vi "DAQ_TDV Meas Configure and Measure.vi"(0 "DAQmx Task In":refnum<k21>, 2 "Execution Settings":T2, 5 "Range and Terminal Settings":T7={"Global Settings"={"Min Range(V)"=-10.0, "Max Range(V)"=10.0, "Terminal Configuration"=10083}, "Specific Channel Settings"=[]} {"Specific Channel Settings"."Terminal Configuration" items=["RSE"=10083, "NRSE"=10078, "Differential"=10106, "Pseudodifferential"=12529]; "Specific Channel Settings"."Max Range" format="%.2p"; "Specific Channel Settings"."Min Range" format="%.2p"; "Global Settings"."Terminal Configuration" items=["RSE"=10083, "NRSE"=10078, "Differential"=10106, "Pseudodifferential"=12529]; "Global Settings"."Max Range(V)" format="%.2p"; "Global Settings"."Min Range(V)" format="%.2p"}, 7 "Timing and Trigger Settings":T4={"Timing Settings"={"Sample Clock Source"="OnboardClock", "Sample Rate(Hz)"=10000.0, "Number of Samples"=1000, "Sample Timing Engine"=enum."Auto"}, "Trigger Settings"={"Trigger Type"=enum."No Trigger", "Digital Start Trigger Source"="", "Digital Start Trigger Edge"=10280}} {"Trigger Settings"."Digital Start Trigger Edge" items=["Rising"=10280, "Falling"=10171]; "Timing Settings"."Sample Rate(Hz)" format="%.2p"}, 9 "Periodic Waveform \nMeasurements?":bool=TRUE, 11 "error in":errorcluster) -> (4 "DAQmx Task Out":refnum<k21>, 6 "Voltage Waveforms":waveform(dbl)[](graph), 8 "Time Domain Measurements":T1 {"Voltage Waveform duty cycle (%)" format="%.2p"; "Voltage Waveform Period (s)" format="%.2p"; "Voltage Frequency(Hz)" format="%.2p"; "Vpp Amplitude(V)" format="%.2p"; "Mean DC Voltage (V)" format="%.2p"}, 10 "Acquisition Time (s)":dbl format="%.2p", 15 "error out":errorcluster)   [LabVIEW 2021, in "DAQ_Time Domain Measurement.lvlib"]
doc: "Configure, initiate and fetch time domain measurements from the channels configured.\n\nNOTE: Captured waveform should contain more than one cycle to calculate Voltage Waveform Period (s) and Voltage Waveform duty cycle (%)."
uses:
  DAQ_Time Domain Measurement.lvlib
  Typedefs/Time Domain Measurements.ctl
  Typedefs/Timing & Trigger Settings.ctl
  Typedefs/Timing Settings.ctl
  Typedefs/Trigger Settings.ctl
  Typedefs/Range and Terminal Settings.ctl
  Typedefs/Specific Channel Settings.ctl
  Typedefs/Execution Settings.ctl
  Common/Typedefs/Execution Options - Measure.ctl
  <vilib>/DAQmx/read.llb/DAQmx Read (Analog 1D Wfm NChan NSamp).vi
  <vilib>/DAQmx/configure/timing.llb/DAQmx Timing (Sample Clock).vi
  <vilib>/DAQmx/configure/trigger.llb/DAQmx Start Trigger (Digital Edge).vi
  <vilib>/DAQmx/miscellaneous.llb/DAQmx Fill In Error Info.vi
  <resource>/objmgr/daqmx.rc
panel:
  # "Outputs"
  # "Inputs"
  # "Measure Settings"
  # "Min. Range(V)"
  # "Max. Range(V)"
  # "Terminal Configuration"
  # "Physical Channel Name"
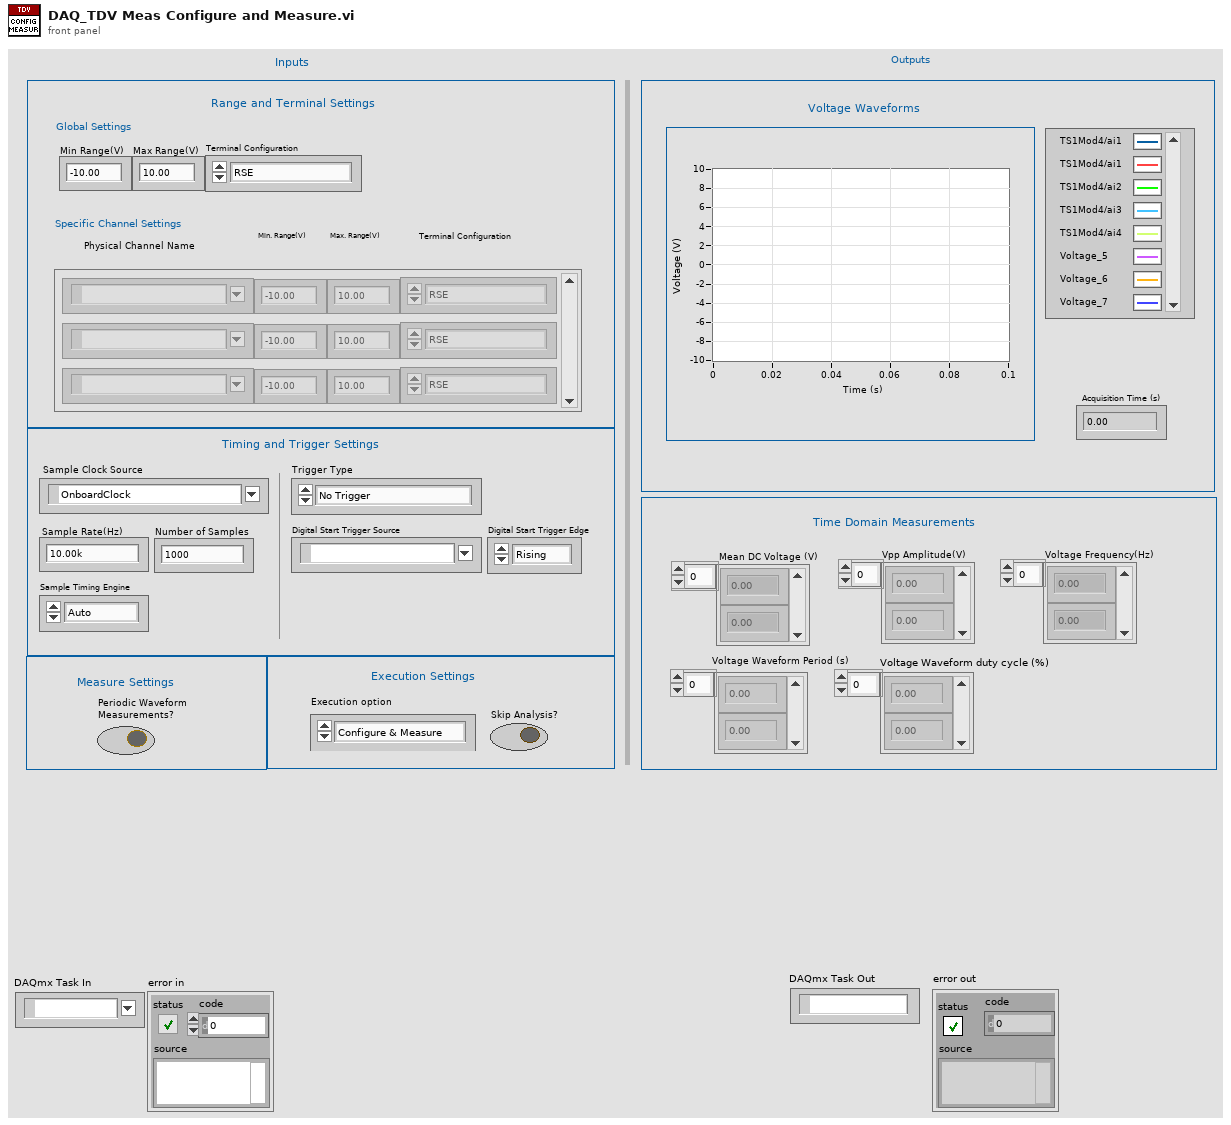
[diagram p1: front panel]
types:
  T1 = typedef "DAQ_Time Domain Measurement.lvlib/Time Domain Measurements.ctl" = cluster{"Mean DC Voltage (V)":dbl[], "Vpp Amplitude(V)":dbl[], "Voltage Frequency(Hz)":dbl[], "Voltage Waveform Period (s)":dbl[], "Voltage Waveform duty cycle (%)":dbl[]}
  T2 = typedef "DAQ_Time Domain Measurement.lvlib/Execution Settings.ctl" = cluster{"Execution option":T3, "Skip Analysis?":bool}
  T3 = typedef "Execution Options - Measure.ctl" = enum16{"Configure & Measure", "Configure only", "Measure only"}
  T4 = typedef "DAQ_Time Domain Measurement.lvlib/Timing & Trigger Settings.ctl" = cluster{"Timing Settings":T5, "Trigger Settings":T6}
  T5 = typedef "DAQ_Time Domain Measurement.lvlib/Timing Settings.ctl" = cluster{"Sample Clock Source":tag, "Sample Rate(Hz)":dbl, "Number of Samples":i32, "Sample Timing Engine":enum16{"te0", "te1", "ai", "Auto"}}
  T6 = typedef "DAQ_Time Domain Measurement.lvlib/Trigger Settings.ctl" = cluster{"Trigger Type":enum16{"No Trigger", "Digital Start"}, "Digital Start Trigger Source":tag, "Digital Start Trigger Edge":i32}
  T7 = typedef "DAQ_Time Domain Measurement.lvlib/Range and Terminal Settings.ctl" = cluster{"Global Settings":cluster{"Min Range(V)":dbl, "Max Range(V)":dbl, "Terminal Configuration":i32}, "Specific Channel Settings":T8[]}
  T8 = typedef "DAQ_Time Domain Measurement.lvlib/Specific Channel Settings.ctl" = cluster{"Active Channels":tag, "Min Range":dbl, "Max Range":dbl, "Terminal Configuration":i32}
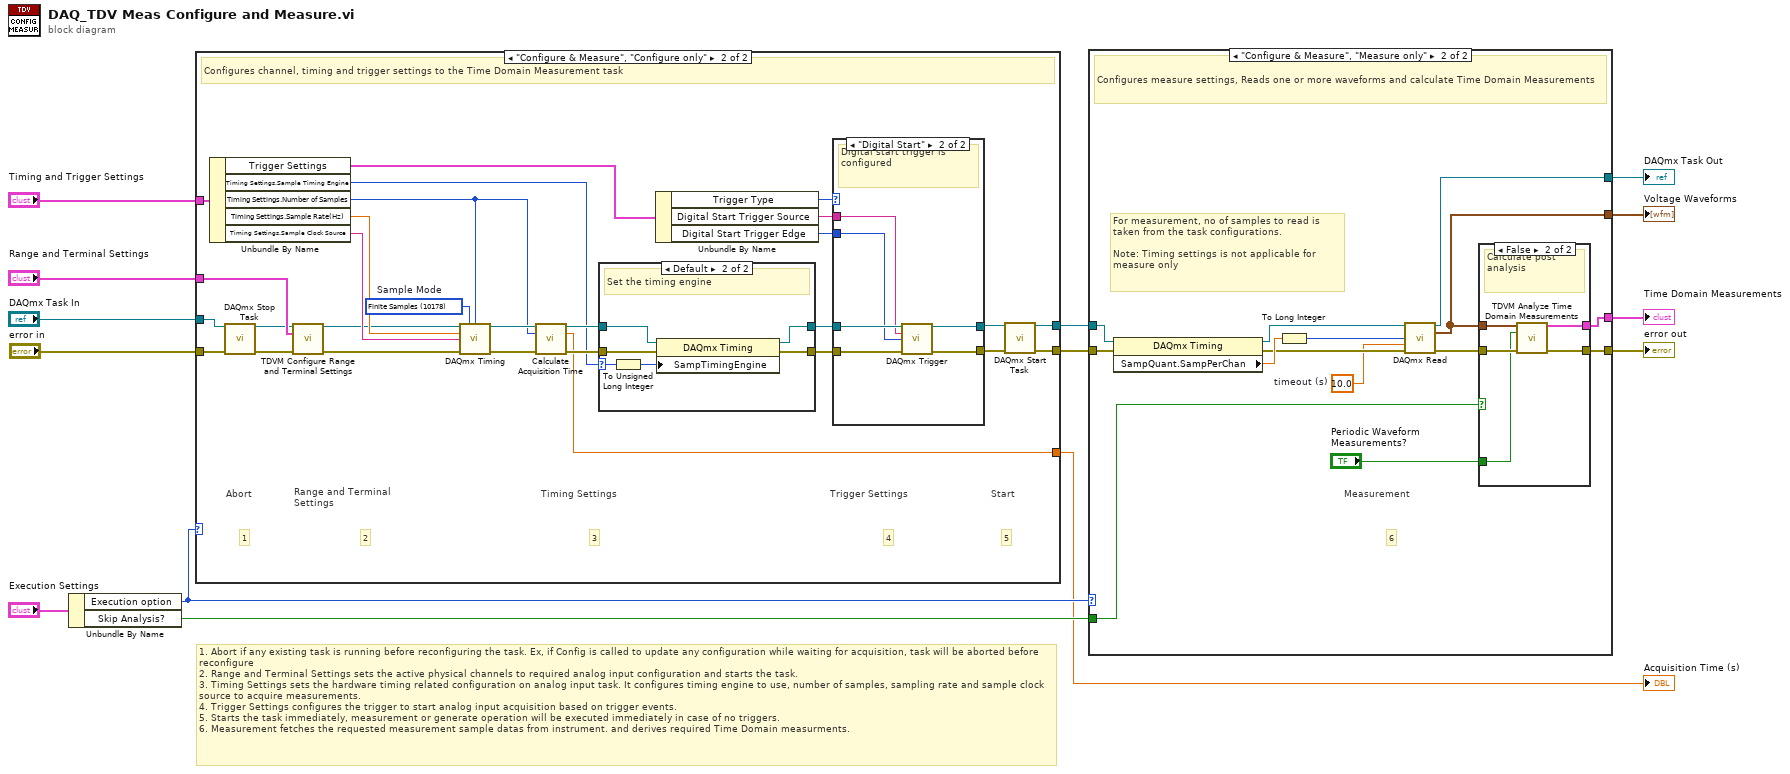
[diagram p0: block diagram]
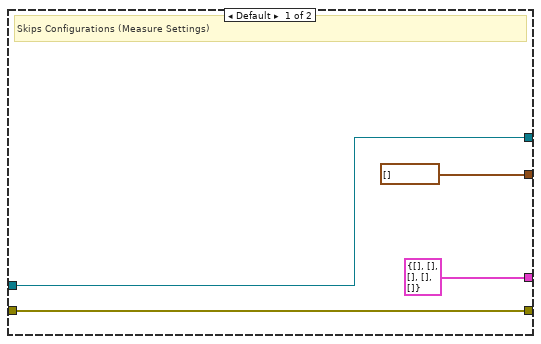
[diagram p5: hidden frame]
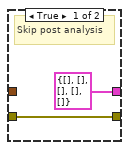
[diagram p6: hidden frame]
diagram:
  # "1. Abort if any existing task is running before reconfiguring the task. Ex, if Config is called to update any configuration while waiting for acquisition, task will be aborted before reconfigure\n2. Range and Terminal Settings sets the active physical channels to required analog input configuration and starts the task.\n3. Timing Settings sets the hardware timing related configuration on analog input task. It configures timing engine to use, number of samples, sampling rate and sample clock source to acquire measurements.\n4. Trigger Settings configures the trigger to start analog input acquisition based on trigger events.\n5. Starts the task immediately, measurement or generate operation will be executed immediately in case of no triggers.\n6. Measurement fetches the requested measurement sample datas from instrument. and derives required Time Domain measurments."
  n1 = Unbundle By Name("Execution Settings") -> ("Execution option"=w3:T3, "Skip Analysis?"=w2:bool)
  n2 = case shown="\"Configure & Measure\", \"Configure only\"" w3 {
    tunnel: "error in" -> [w16 w20]
    tunnel: "DAQmx Task In" -> [w15 w22]
    tunnel: "Timing and Trigger Settings" -> [_ w38]
    tunnel: [w15 w18] -> w13
    tunnel: [w16 w32] -> w14
    tunnel: "Range and Terminal Settings" -> [_ w25]
    tunnel: [_ w17] -> w1
    frame Default {
      # "Skips Configurations (Channel, Timing and Trigger Settings)"
    }
    frame "Configure & Measure", "Configure only" {
      w42 = 10178 items=["Finite Samples"=10178, "Continuous Samples"=10123, "Hardware Timed Single Point"=12522]  # Sample Mode
      # "1"
      # "Abort"
      # "5"
      # "Start"
      # "4"
      # "3"
      # "2"
      # "Range and Terminal \nSettings"
      # "Trigger Settings"
      # "Timing Settings"
      # "Configures channel, timing and trigger settings to the Time Domain Measurement task"
      n3 = Unbundle By Name(w38) -> ("Trigger Settings"=w24:T6, "Timing Settings.Sample Timing Engine"=w33:enum16{"te0", "te1", "ai", "Auto"}, "Timing Settings.Number of Samples"=w31:i32, "Timing Settings.Sample Rate(Hz)"=w39:dbl, "Timing Settings.Sample Clock Source"=w40:tag)
      n4 = call <vilib>:"DAQmx Stop Task.vi"("task/channels in"=w22, "error in"=w20) -> ("task out"=w23:refnum<k21>, "error out"=w21:errorcluster)  [unwired: 12 in]
      n5 = call "TDVM Configure Range and Terminal Settings.vi"("DAQmx Task In"=w23, "Range and Terminal Settings"=w25, "error in (no error)"=w21) -> ("DAQmx Task Out"=w26:refnum<k21>, "error out"=w27:errorcluster)  [unwired: 11 in]
      n6 = call-poly <vilib>:"DAQmx Timing.vi"("task/channels in"=w26, "sample mode"=w42, "samples per channel"=w31, "rate"=w39, "source"=w40, "error in"=w27) -> ("task out"=w44:refnum<k21>, "error out"=w43:errorcluster)  [unwired: 8 in]
      n7 = call "Calculate Acquisition Time.vi"("Refnum in"=w44, "Number of Samples"=w31, "error in (no error)"=w43) -> ("Refnum out"=w35:refnum<k21>, "Acquisition Time Period (s)"=w17:dbl, "error out"=w41:errorcluster)  [unwired: 10 in]
      n8 = case shown="Default" w33 {
        selector: w33 -> [_ w48]
        tunnel: w41 -> [w46 w52]
        tunnel: [w46 w51] -> w36
        tunnel: w35 -> [w45 w50]
        tunnel: [w45 w49] -> w34
        frame "Auto" {
          # "Timing engine is auto-selected"
        }
        frame Default {
          # "Set the timing engine"
          n9 = To Unsigned Long Integer(number=w48) -> (unsigned 32bit integer=w47:u32)
          n10 = property class="DAQmx Timing"(reference=w50, error in=w52, "SampTimingEngine"=w47) -> (reference out=w49:refnum<k21>, error out=w51:errorcluster)
        }
      }
      n11 = Unbundle By Name(w24) -> ("Trigger Type"=w28:enum16{"No Trigger", "Digital Start"}, "Digital Start Trigger Source"=w30:tag, "Digital Start Trigger Edge"=w29:i32)
      n12 = case shown="\"Digital Start\"" w28 {
        tunnel: w34 -> [w54 w60]
        tunnel: w36 -> [w53 w59]
        tunnel: [w54 w58] -> w19
        tunnel: [w53 w57] -> w37
        tunnel: w30 -> [_ w56]
        tunnel: w29 -> [_ w55]
        frame Default {
          # "No Trigger settings has been configured"
        }
        frame "Digital Start" {
          # "Digital start trigger is configured"
          n13 = call-poly <vilib>:"DAQmx Trigger.vi"("task/channels in"=w60, "source"=w56, "edge"=w55, "error in"=w59) -> ("task out"=w58:refnum<k21>, "error out"=w57:errorcluster)  [unwired: 10 in]
        }
      }
      n14 = call <vilib>:"DAQmx Start Task.vi"("task/channels in"=w19, "error in"=w37) -> ("task out"=w18:refnum<k21>, "error out"=w32:errorcluster)  [unwired: 12 in]
    }
  }
  "Acquisition Time (s)" <- w1
  n15 = case shown="\"Configure & Measure\", \"Measure only\"" w3 {
    tunnel: w13 -> [w64 w74]
    tunnel: w14 -> [w63 w71]
    tunnel: [w64 w76] -> w12
    tunnel: [w63 w78] -> w10
    tunnel: [T1 {"Mean DC Voltage (V)"=[], "Vpp Amplitude(V)"=[], "Voltage Frequency(Hz)"=[], "Voltage Waveform Period (s)"=[], "Voltage Waveform duty cycle (%)"=[]} ("DC Measurements") w69] -> w6
    tunnel: [waveform(dbl)[] [] ("data") w68] -> w5
    tunnel: w2 -> [_ w66]
    frame Default {
      # "Skips Configurations (Measure Settings)"
    }
    frame "Configure & Measure", "Measure only" {
      w67 = 10.0  # timeout (s)
      # "For measurement, no of samples to read is taken from the task configurations.\n\nNote: Timing settings is not applicable for measure only"
      # "6"
      # "Measurement"
      # "Configures measure settings, Reads one or more waveforms and calculate Time Domain Measurements"
      n16 = property class="DAQmx Timing"(reference=w74, error in=w71) -> (reference out=w75:refnum<k21>, error out=w72:errorcluster, "SampQuant.SampPerChan"=w73:dbl)
      n17 = To Long Integer(number=w73) -> (32bit integer=w70:i32)
      n18 = call-poly <vilib>:"DAQmx Read.vi"("task/channels in"=w75, "number of samples per channel"=w70, "timeout"=w67, "error in"=w72) -> ("task out"=w76:refnum<k21>, "data"=w68:waveform(dbl)[], "error out"=w77:errorcluster)  [unwired: 9 in]
      n19 = case shown="False" w66 {
        tunnel: w68 -> [_ w85]
        tunnel: [w80 w84] -> w78
        tunnel: w77 -> [w80 w83]
        tunnel: [T1 {"Mean DC Voltage (V)"=[], "Vpp Amplitude(V)"=[], "Voltage Frequency(Hz)"=[], "Voltage Waveform Period (s)"=[], "Voltage Waveform duty cycle (%)"=[]} ("DC Measurements") w82] -> w69
        tunnel: "Periodic Waveform \nMeasurements?" -> [_ w81]
        frame True {
          # "Skip post analysis"
        }
        frame False {
          # "Calculate post analysis"
          n20 = call "TDVM Analyze Time Domain Measurements.vi"("Voltage Waveforms In"=w85, "Periodic Waveform \nMeasurements"=w81, "error in (no error)"=w83) -> ("Time Domain Measurements"=w82:T1, "error out"=w84:errorcluster)  [unwired: 11 in]
        }
      }
    }
  }
  "error out" <- w10
  "DAQmx Task Out" <- w12
  "Time Domain Measurements" <- w6
  "Voltage Waveforms" <- w5
